vi "Handle Last Ack Core.vi"(4 "error in":errorcluster, 6 "Last Ack":refnum<class "Last Ack.lvclass">, 7 "CRIO MSS Test Actor in":refnum<class "MSS Target Actor.lvclass">) -> (0 "error out":errorcluster, 3 "CRIO MSS Test Actor out":refnum<class "MSS Target Actor.lvclass">)   [LabVIEW 2023, in "MSS Target Actor.lvlib" / "MSS Target Actor.lvclass"]
doc: "(<B>Filename</B>: Actor Framework.lvlib:Actor.lvclass:Handle Last Ack Core.vi)\n\nDefines how the caller actor responds to the Last Ack message from a nested actor. The Last Ack message is the final message a nested actor sends to its caller before it shuts down. The message contains information about the final state of the nested actor.\n\nBy default, this method does nothing except return any error the nested actor sent. A descendant class may override this method to define behavior."
uses:
  MSS Target Actor.lvclass
  <vilib>/ActorFramework/LastAck/Last Ack.lvclass
  <vilib>/ActorFramework/LastAck/Last Ack.lvclass/Last Ack.ctl
  MSS Target Actor.lvclass/MSS Target Actor.ctl
  <vilib>/ActorFramework/Actor/Actor.lvclass
  C:/Program Files/National Instruments/LabVIEW 2023/vi.lib/ActorFramework/Actor/Actor.lvclass
  D:/git/HAL/HAL GOOP4/MSS Target/MSS Target Actor/MSS Target Actor.lvclass
  D:/git/HAL/HAL GOOP4/MSS Target/IMSS Target Actor/IMSS Target Actor.lvclass
  C:/Program Files/National Instruments/LabVIEW 2023/vi.lib/ni/Actors/Network Endpoint Actors/Nested Endpoint Caller/Nested Endpoint Caller/Nested Endpoint Caller.lvclass
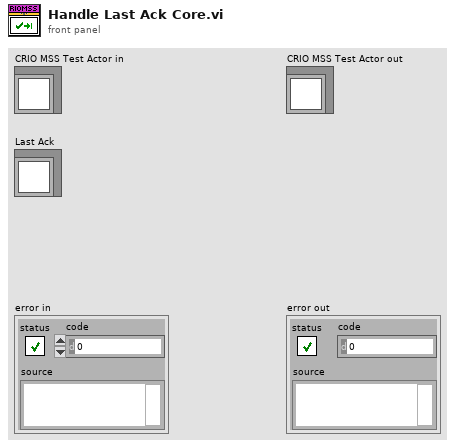
[diagram p1: front panel]
types:
  T1 = map{string, refnum<class "Message Enqueuer.lvclass">}
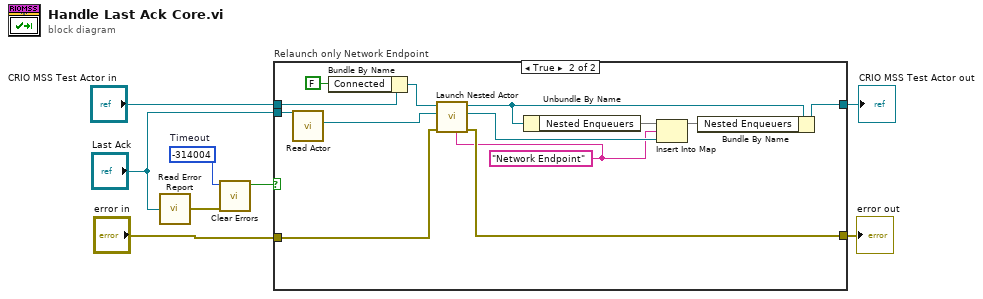
[diagram p0: block diagram]
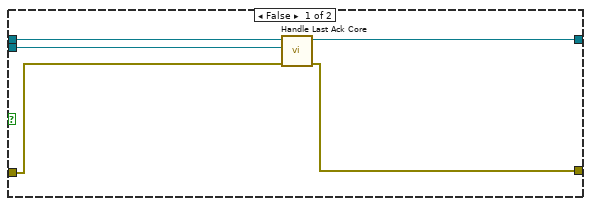
[diagram p2: hidden frame]
diagram:
  w7 = -314004  # Timeout
  n1 = call <vilib>:"Read Error Report.vi"("Last Ack"="Last Ack") -> ("error report"=w8:errorcluster)
  n2 = call <vilib>:"Clear Errors.vi"("error in (no error)"=w8, "specific error code to clear (0: all)"=w7) -> ("specific error cleared?"=w6:bool)  [unwired: 4 in, 1 out]
  n3 = case "Relaunch only Network Endpoint" shown="True" w6 {
    tunnel: "CRIO MSS Test Actor in" -> [w13 w16]
    tunnel: [w11 w26] -> w4
    tunnel: [w12 w22] -> w5
    tunnel: "Last Ack" -> [w10 w19]
    tunnel: "error in" -> [w9 w17]
    frame False {
      n4 = call-parent "Handle Last Ack Core.vi"("error in (no error)"=w9, "Last Ack"=w10, "Actor in"=w13) -> ("error out"=w11:errorcluster, "Actor out"=w12:refnum<class "MSS Target Actor.lvclass">)  [unwired: 3 in]
    }
    frame True {
      w20 = "Network Endpoint" ("key")
      n5 = call <vilib>:"Read Actor.vi"("Last Ack"=w19) -> ("Actor"=w18:refnum<class "Actor.lvclass">)  [unwired: 10 in]
      n6 = Bundle By Name(cluster=w16, "Connected"=FALSE) -> (w15:refnum<class "MSS Target Actor.lvclass">)
      n7 = call <vilib>:"Launch Nested Actor.vi"("Debug Alias"=w20, "error in (no error)"=w17, "Nested Actor"=w18, "Caller Actor in"=w15) -> ("error out"=w26:errorcluster, "Nested Actor's Enqueuer"=w23:refnum<class "Message Enqueuer.lvclass">, "Caller Actor in"=w25:refnum<class "MSS Target Actor.lvclass">)  [unwired: 5 in]
      n8 = Unbundle By Name(w25) -> ("Nested Enqueuers"=w24:T1)
      n9 = Insert Into Map(map in=w24, key=w20, value=w23) -> (map out=w21:T1)  [unwired: 2 out]
      n10 = Bundle By Name(cluster=w25, "Nested Enqueuers"=w21) -> (w22:refnum<class "MSS Target Actor.lvclass">)
    }
  }
  "CRIO MSS Test Actor out" <- w5
  "error out" <- w4
